vi "Add Quotes for String Input Database.vi"(11 "String in":string) -> (3 "String Out":string)   [LabVIEW 2020]
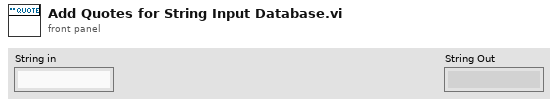
[diagram p1: front panel]
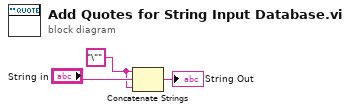
[diagram p0: block diagram]
diagram:
  w2 = "\"" ("string")
  n1 = Concatenate Strings(w2, "String in", w2) -> (→"String Out":string)
